vi "scan position (SubVI).vi"(6 "字符串":string, 9 "queue out输入":refnum<queue>, 11 "队列输入":refnum<queue>) -> (0 "错误输出":errorcluster)   [LabVIEW 2019, in "SubVI.lvlib"]
uses:
  SubVI.lvlib
  config.ctl
  Instrument.ctl
  lib/QDInstrument.dll
panel:
  # "(真是通道1，假是通道2)"
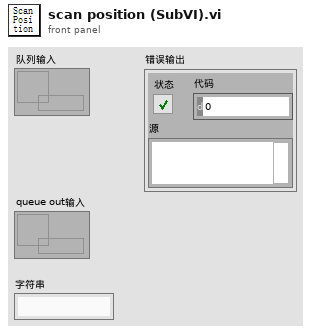
[diagram p1: front panel]
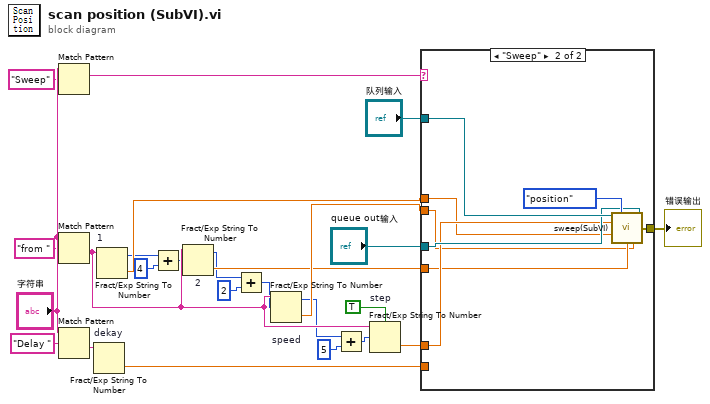
[diagram p0: block diagram]
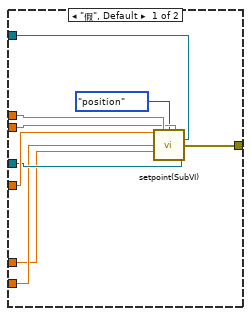
[diagram p2: hidden frame]
diagram:
  n1 = Match Pattern(string="字符串", regular expression="Sweep" ("正则表达式")) -> (match substring=w13:string)  [unwired: 1 in, 3 out]
  n2 = Match Pattern(string="字符串", regular expression="from " ("正则表达式")) -> (after substring=w17:string)  [unwired: 1 in, 3 out]
  n3 = Match Pattern(string="字符串", regular expression="Delay " ("正则表达式")) -> (after substring=w16:string)  [unwired: 1 in, 3 out]
  n4 = Fract/Exp String To Number "dekay"(string=w16) -> (number=w19:dbl)  [unwired: 3 in, 1 out]
  n5 = Fract/Exp String To Number "1"(string=w17) -> (offset past number=w2:i32, number=w24:dbl)  [unwired: 3 in]
  n6 = Add(x=w2, y=4) -> (x+y=w4:i32)
  n7 = Fract/Exp String To Number "2"(string=w17, offset=w4) -> (offset past number=w5:i32, number=w18:dbl)  [unwired: 2 in]
  n8 = Add(x=w5, y=2) -> (x+y=w7:i32)
  n9 = Fract/Exp String To Number "speed"(string=w17, offset=w7) -> (offset past number=w8:i32, number=w21:dbl)  [unwired: 2 in]
  n10 = Add(x=w8, y=5) -> (x+y=w10:i32)
  n11 = Fract/Exp String To Number "step"(use system decimal point (T)=TRUE ("使用系统小数点(T)"), string=w17, offset=w10) -> (number=w20:dbl)  [unwired: 1 in, 1 out]
  n12 = case shown="\"Sweep\"" w13 {
    tunnel: w18 -> [w34 w37]
    tunnel: w19 -> [w30 _]
    tunnel: w20 -> [w29 w39]
    tunnel: w21 -> [w28 w36]
    tunnel: "queue out输入" -> [w32 w40]
    tunnel: "队列输入" -> [w31 w42]
    tunnel: w24 -> [w33 w38]
    tunnel: [w26 w35] -> w25
    frame "假", Default {
      n13 = call "setpoint(SubVI).vi"("Filed 2"=w34, "Field"=w33, "类型"=enum16{"temp", "field", "position"}."position", "Rate/speed"=w28, "data"=w31, "Delay"=w30, "steps number"=w29, "config"=w32) -> ("错误输出"=w26:errorcluster)  [unwired: 7 in]
    }
    frame "Sweep" {
      n14 = call "sweep(SubVI).vi"("data"=w42, "类型"=enum16{"temp", "field", "position"}."position", "config"=w40, "steps number"=w39, "Field"=w38, "Field 2"=w37, "Rate、speed"=w36) -> ("错误输出"=w35:errorcluster)  [unwired: 8 in]
    }
  }
  "错误输出" <- w25
